vi "Read kickZ.vi"(8 "error in (no error)":errorcluster, 11 "KickToSkill_v2 in":refnum<class "KickToSkill_v2.lvclass">) -> (0 "error out":errorcluster, 2 "kickZ":dbl, 3 "KickToSkill_v2 out":refnum<class "KickToSkill_v2.lvclass">)   [LabVIEW 2023, in "KickToSkill_v2.lvclass"]
uses:
  KickToSkill_v2.lvclass
  KickToSkill_v2.lvclass/KickToSkill_v2.ctl
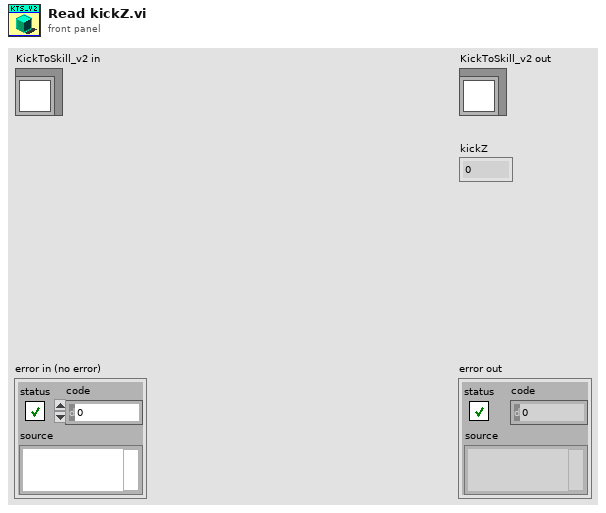
[diagram p1: front panel]
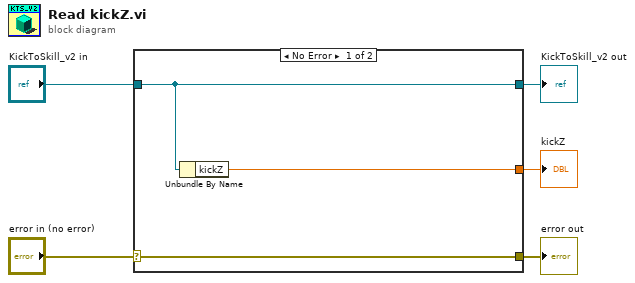
[diagram p0: block diagram]
diagram:
  n1 = case shown="No Error" "error in (no error)" {
    selector: "error in (no error)" -> [w8 w9]
    tunnel: [w8 w9] -> w4
    tunnel: [w7 w10] -> w2
    tunnel: "KickToSkill_v2 in" -> [w7 w10]
    tunnel: [w6 _] -> w1
    frame No Error {
      n2 = Unbundle By Name(w7) -> ("kickZ"=w6:dbl)
    }
    frame Error {
    }
  }
  "error out" <- w4
  "KickToSkill_v2 out" <- w2
  "kickZ" <- w1
